vi "复件 复件 数组求和  雷-9.vi"() -> (0 "数组 2":i16[][](array[numeric]))   [LabVIEW 2014]
panel:
  out "数组":dbl[][](array[numeric])
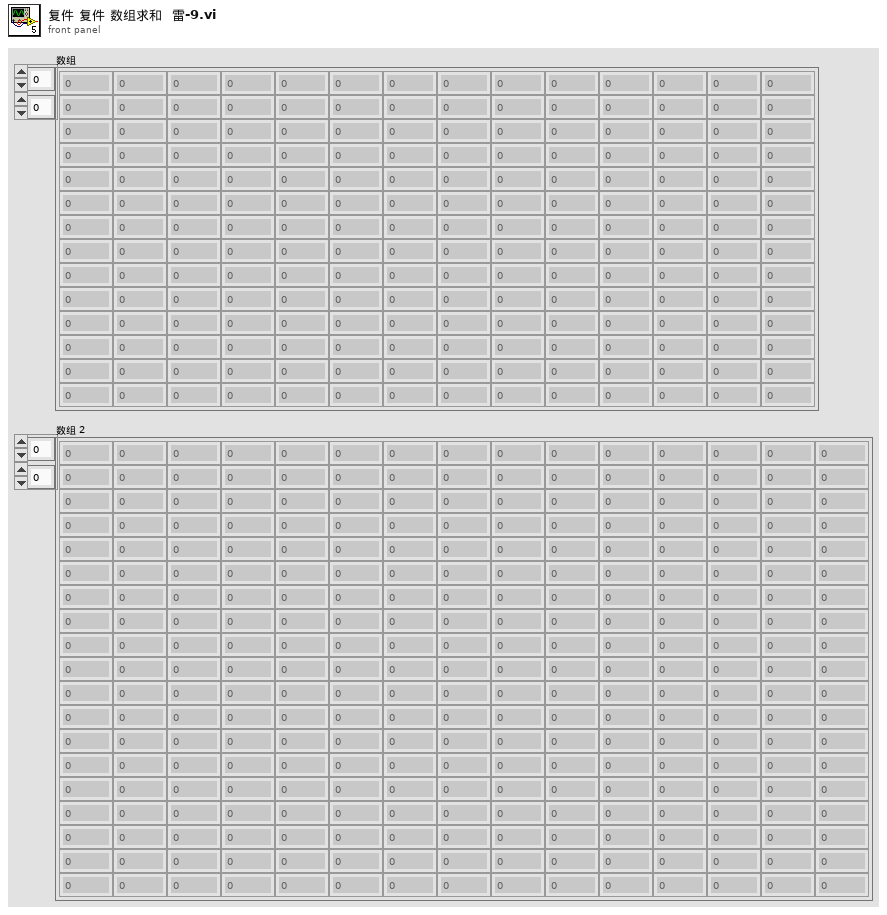
[diagram p1: front panel]
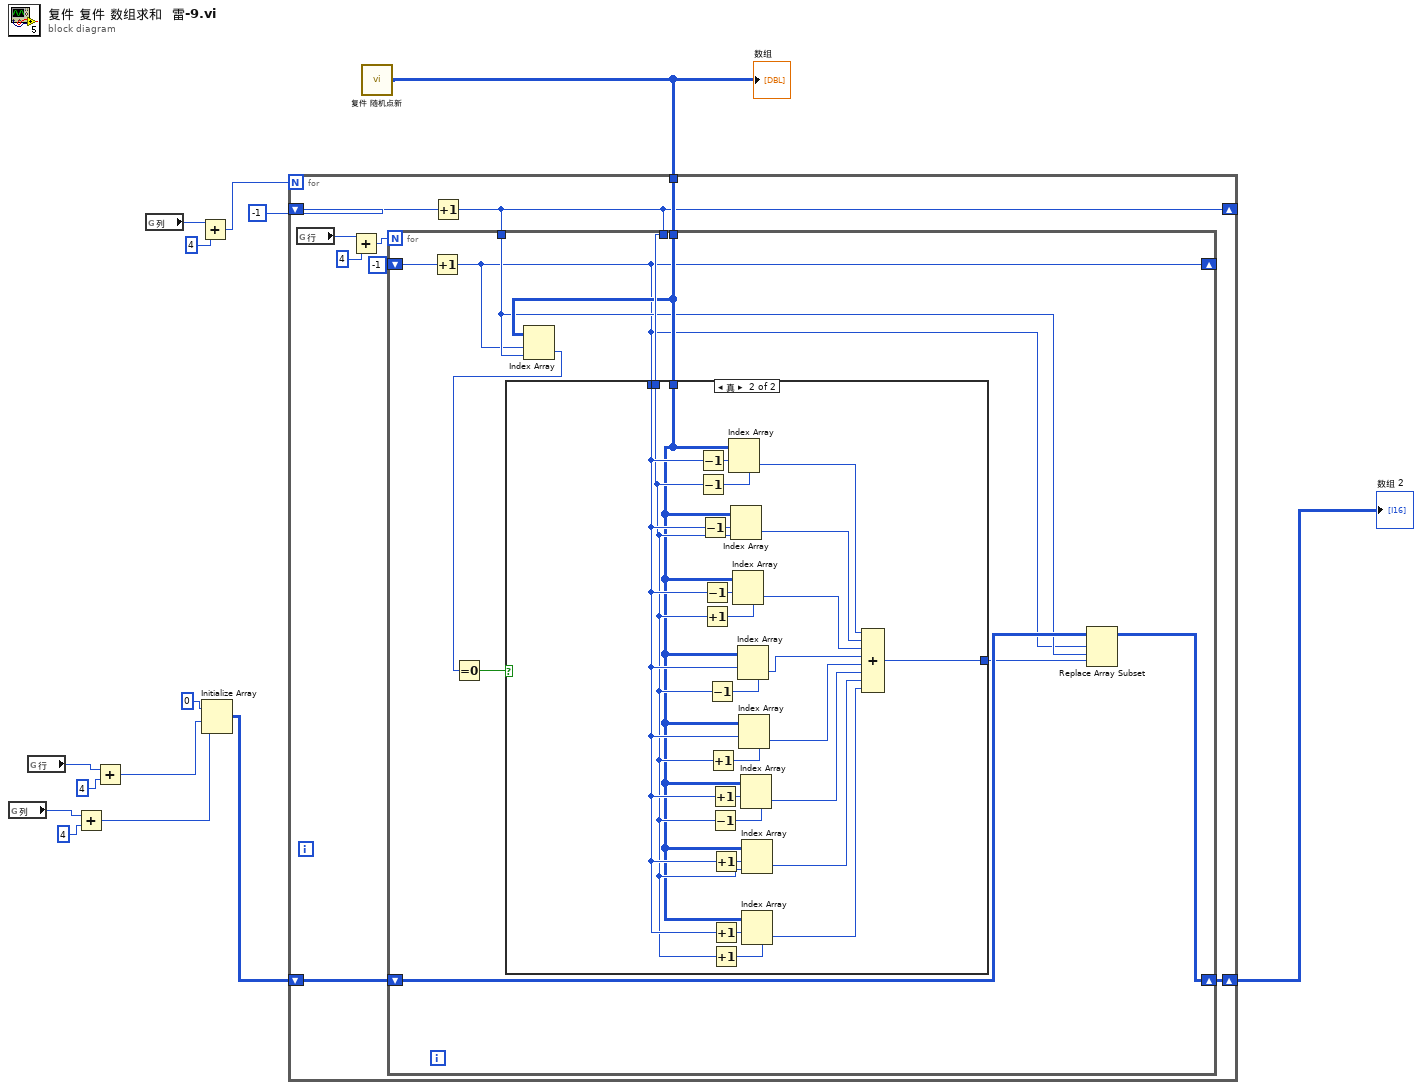
[diagram p0: block diagram]
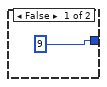
[diagram p2: hidden frame]
diagram:
  n1 = global read "全局 1.vi" "列"() -> (w5:i32)
  n2 = global read "全局 1.vi" "行"() -> (w7:i32)
  n3 = Add(x=w5, y=4) -> (x+y=w3:i32)
  n4 = Add(x=w7, y=4) -> (x+y=w4:i32)
  n5 = global read "全局 1.vi" "列"() -> (w12:i32)
  n6 = Add(x=w12, y=4) -> (x+y=w10:i32)
  n7 = Initialize Array(0, w4, w3) -> (w2:i32[][])
  n8 = call "复件 随机点新.vi"() -> ("输出数组"=w13:i32[][])
  "数组" <- w13
  n9 = for {
    N: w10 -> [_]
    shift-right: [w20] -> _
    shift-left: -1 -> [w23]
    tunnel: w13 -> [w21]
    shift-right: [w15] -> w1
    shift-left: w2 -> [w16]
    n10 = global read "全局 1.vi" "行"() -> (w19:i32)
    n11 = Add(x=w19, y=4) -> (x+y=w17:i32)
    n12 = Increment(x=w23) -> (x+1=w20:i32)
    n13 = for {
      N: w17 -> [_]
      shift-right: [w25] -> _
      shift-left: -1 -> [w33]
      tunnel: w20 -> [w32]
      tunnel: w21 -> [w31]
      tunnel: w20 -> [w26]
      shift-right: [w24] -> w15
      shift-left: w16 -> [w28]
      n14 = Increment(x=w33) -> (x+1=w25:i32)
      n15 = Index Array(array=w31, index (row)=w25, index (col)=w26) -> (element=w29:i32)
      n16 = Equal To 0?(x=w29) -> (x = 0?=w30:bool)
      n17 = case shown="真" w30 {
        tunnel: w25 -> [_ w46]
        tunnel: w32 -> [_ w45]
        tunnel: w31 -> [_ w44]
        tunnel: [9 w35] -> w27
        frame False {
        }
        frame True {
          n18 = Decrement(x=w46) -> (x-1=w58:i32)
          n19 = Decrement(x=w45) -> (x-1=w57:i32)
          n20 = Decrement(x=w46) -> (x-1=w56:i32)
          n21 = Decrement(x=w46) -> (x-1=w54:i32)
          n22 = Increment(x=w45) -> (x+1=w55:i32)
          n23 = Decrement(x=w45) -> (x-1=w53:i32)
          n24 = Increment(x=w45) -> (x+1=w52:i32)
          n25 = Increment(x=w46) -> (x+1=w51:i32)
          n26 = Decrement(x=w45) -> (x-1=w50:i32)
          n27 = Increment(x=w46) -> (x+1=w49:i32)
          n28 = Increment(x=w46) -> (x+1=w48:i32)
          n29 = Increment(x=w45) -> (x+1=w47:i32)
          n30 = Index Array(array=w44, index (row)=w58, index (col)=w57) -> (element=w43:i32)
          n31 = Index Array(array=w44, index (row)=w56, index (col)=w45) -> (element=w42:i32)
          n32 = Index Array(array=w44, index (row)=w54, index (col)=w55) -> (element=w41:i32)
          n33 = Index Array(array=w44, index (row)=w46, index (col)=w53) -> (element=w40:i32)
          n34 = Index Array(array=w44, index (row)=w46, index (col)=w52) -> (element=w39:i32)
          n35 = Index Array(array=w44, index (row)=w51, index (col)=w50) -> (element=w38:i32)
          n36 = Index Array(array=w44, index (row)=w49, index (col)=w45) -> (element=w37:i32)
          n37 = Index Array(array=w44, index (row)=w48, index (col)=w47) -> (element=w36:i32)
          n38 = Compound Arithmetic op=ADD(w43, w42, w41, w40, w39, w38, w37, w36) -> (w35:i32)
        }
      }
      n39 = Replace Array Subset(array=w28, new element=w27, index (row)=w25, index (col)=w26) -> (w24:i32[][])
    }
  }
  "数组 2" <- w1
